vi "Disabled_Default.vi"   [LabVIEW 2014]
uses:
  Global Var.vi
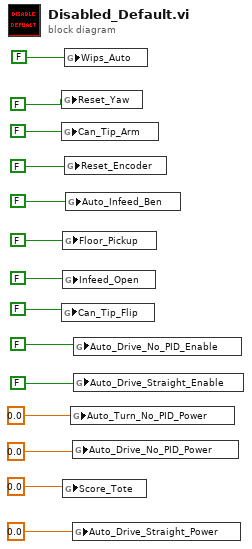
[diagram p0: block diagram]
diagram:
  n1 = global write "Global Var.vi" "Reset_Yaw"(FALSE ("Reset_Yaw")) -> ()
  n2 = global write "Global Var.vi" "Can_Tip_Arm"(FALSE ("Can_Tip_Arm")) -> ()
  n3 = global write "Global Var.vi" "Can_Tip_Flip"(FALSE ("Can_Tip_Flip")) -> ()
  n4 = global write "Global Var.vi" "Floor_Pickup"(FALSE ("Floor_Pickup")) -> ()
  n5 = global write "Global Var.vi" "Infeed_Open"(FALSE ("Infeed_Open")) -> ()
  n6 = global write "Global Var.vi" "Score_Tote"(0.0 ("Score_Tote")) -> ()
  n7 = global write "Global Var.vi" "Wips_Auto"(FALSE ("Reset_Yaw")) -> ()
  n8 = global write "Global Var.vi" "Reset_Encoder"(FALSE ("Reset_Encoder")) -> ()
  n9 = global write "Global Var.vi" "Auto_Infeed_Ben"(FALSE ("Auto_Infeed_Ben")) -> ()
  n10 = global write "Global Var.vi" "Auto_Turn_No_PID_Power"(0.0 ("Auto_Turn_No_PID_Power")) -> ()
  n11 = global write "Global Var.vi" "Auto_Drive_No_PID_Power"(0.0 ("Auto_Drive_No_PID_Power")) -> ()
  n12 = global write "Global Var.vi" "Auto_Drive_Straight_Power"(0.0 ("Auto_Drive_Straight_Power")) -> ()
  n13 = global write "Global Var.vi" "Auto_Drive_No_PID_Enable"(FALSE ("Auto_Drive_No_PID_Enable")) -> ()
  n14 = global write "Global Var.vi" "Auto_Drive_Straight_Enable"(FALSE ("Auto_Drive_Straight_Enable")) -> ()
